vi "Select Drive Mode.vi"   [LabVIEW 2012]
uses:
  Controls/Drive System Mode.ctl
  <vilib>/Rock Robotics/WPI/Joystick/WPI_JoystickGetSetRefNum.vi
  Autonomous/Auto Drive Emulation.vi
  Globals/DriveSystemMode.vi
types:
  T1 = typedef "WPI_JoystickDevRef.ctl" = cluster{"Device":T2}
  T2 = typedef "WPI_JoystickDeviceEnum.ctl" = enum16{"USB 1", "USB 2", "USB 3", "USB 4", "Kinect 1", "Kinect 2"}
  T3 = typedef "Drive System Mode.ctl" = enum16{"Normal", "Crab", "Shoot"}
  T4 = typedef "WPI_JoystickButtonState.ctl" = cluster{"Button 1":bool, "Button 2":bool, "Button 3":bool, "Button 4":bool, "Button 5":bool, "Button 6":bool, "Button 7":bool, "Button 8":bool, "Button 9":bool, "Button 10":bool, "Button 11":bool, "Button 12":bool}
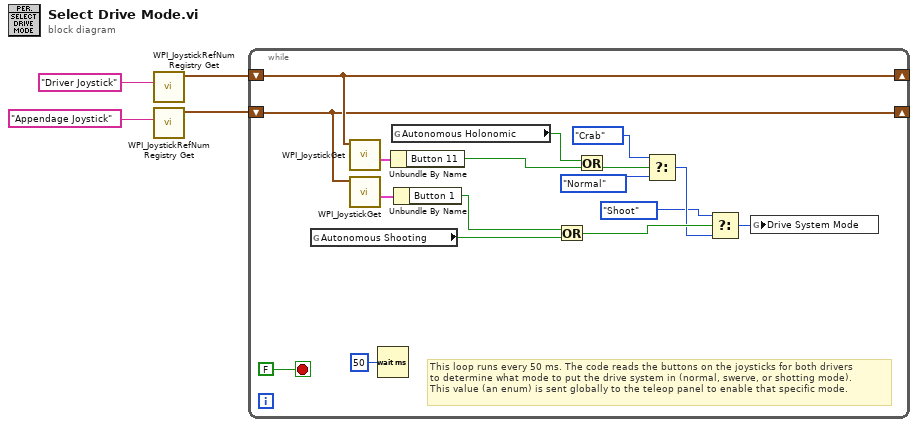
[diagram p0: block diagram]
diagram:
  n1 = call <vilib>:"WPI_JoystickRefNum Registry Get.vi"("refnum name"="Driver Joystick") -> ("JoystickDevRef"=w4:T1)  [unwired: 1 in, 9 out]
  n2 = call <vilib>:"WPI_JoystickRefNum Registry Get.vi"("refnum name"="Appendage Joystick") -> ("JoystickDevRef"=w2:T1)  [unwired: 1 in, 9 out]
  n3 = while {
    shift-right: [w18] -> _
    shift-left: w2 -> [w18]
    shift-right: [w19] -> _
    shift-left: w4 -> [w19]
    stop <- FALSE stop-if-true
    # "This loop runs every 50 ms. The code reads the buttons on the joysticks for both drivers\nto determine what mode to put the drive system in (normal, swerve, or shotting mode).\nThis value (an enum) is sent globally to the teleop panel to enable that specific mode."
    n4 = global read "Auto Drive Emulation.vi" "Autonomous Shooting"() -> (w7:bool)
    n5 = call <vilib>:"WPI_JoystickGet.vi"("JoystickDevRef"=w19) -> ("Buttons"=w17:T4)  [unwired: 4 in, 2 out]
    n6 = call <vilib>:"WPI_JoystickGet.vi"("JoystickDevRef"=w18) -> ("Buttons"=w16:T4)  [unwired: 4 in, 2 out]
    n7 = Wait (ms)(milliseconds to wait=u32 50) -> ()  [unwired: 1 out]
    n8 = Unbundle By Name(w17) -> ("Button 11"=w15:bool)
    n9 = global read "Auto Drive Emulation.vi" "Autonomous Holonomic"() -> (w5:bool)
    n10 = Unbundle By Name(w16) -> ("Button 1"=w14:bool)
    n11 = Or(x=w14, y=w7) -> (x .or. y?=w13:bool)
    n12 = Or(x=w5, y=w15) -> (x .or. y?=w6:bool)
    n13 = Select(t=Drive_System_Mode."Crab" ("Drive System Mode"), s=w6, f=Drive_System_Mode."Normal" ("Drive System Mode")) -> (s? t:f=w12:T3)
    n14 = Select(t=Drive_System_Mode."Shoot" ("Drive System Mode"), s=w13, f=w12) -> (s? t:f=w11:T3)
    n15 = global write "DriveSystemMode.vi" "Drive System Mode"(w11) -> ()
  }
